vi "State XMove.vi"(6 "n":i32, 8 "error in (no error)":errorcluster, 10 "Lua to in":refnum<class "Lua.lvclass">, 11 "Lua from in":refnum<class "Lua.lvclass">) -> (0 "error out":errorcluster, 2 "Lua to out":refnum<class "Lua.lvclass">, 3 "Lua from out":refnum<class "Lua.lvclass">)   [LabVIEW 2020, in "Lua for LabVIEW.lvlib" / "Lua.lvclass"]
doc: "Starts and resumes a coroutine in the given thread L.\n\nTo start a coroutine, you push onto the thread stack the main function plus any arguments; then you call lua_resume, with nargs being the number of arguments. This call returns when the coroutine suspends or finishes its execution. When it returns, the stack contains all values passed to lua_yield, or all values returned by the body function. lua_resume returns LUA_YIELD if the coroutine yields, LUA_OK if the coroutine finishes its execution without errors, or an error code in case of errors (see lua_pcall).\n\nIn case of errors, the stack is not unwound, so you can use the debug API over it. The error object is on the top of the stack.\n\nTo resume a coroutine, you remove any results from the last lua_yield, put on its stack only the values to be passed as results from yield, and then call lua_resume.\n\nThe parameter from represents the coroutine that is resuming L. If there is no such coroutine, this parameter can be NULL."
uses:
  Lua.lvclass
  Lua.lvclass/Lua.ctl
  lib/lua.dll/lua.dll.lvlib
  lib/lua.dll/lua_thread_status.ctl
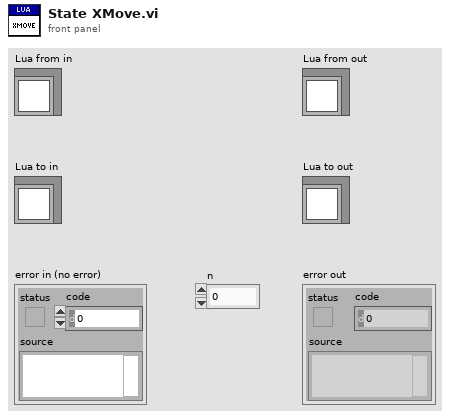
[diagram p1: front panel]
types:
  T1 = typedef "lua.dll.lvlib/lua_thread_status.ctl" = enum8{"LUA_OK", "LUA_YIELD", "LUA_ERRRUN", "LUA_ERRSYNTAX", "LUA_ERRMEM", "LUA_ERRERR"}
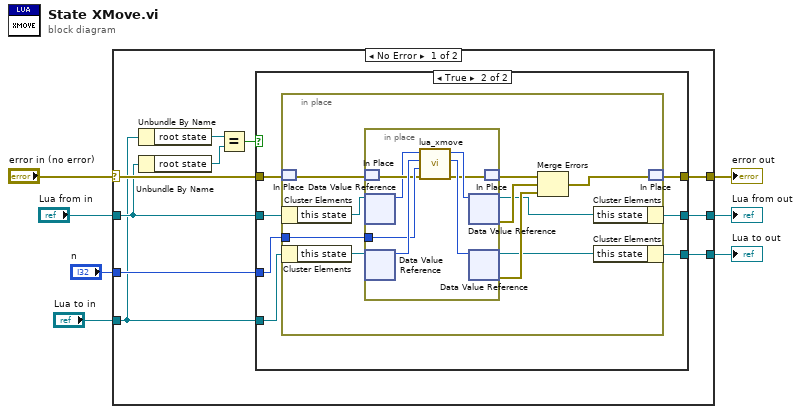
[diagram p0: block diagram]
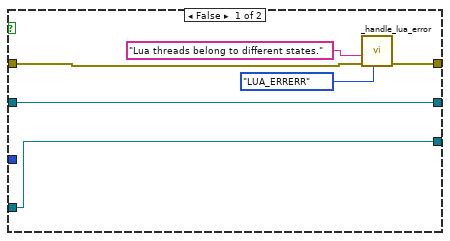
[diagram p2: hidden frame]
diagram:
  n1 = case shown="No Error" "error in (no error)" {
    selector: "error in (no error)" -> [w15 w50]
    tunnel: [w16 w50] -> w4
    tunnel: [w17 w49] -> w7
    tunnel: "Lua from in" -> [w13 w49]
    tunnel: "n" -> [w14 _]
    tunnel: "Lua to in" -> [w8 w48]
    tunnel: [w9 w48] -> w1
    frame No Error {
      n2 = Unbundle By Name(w8) -> ("root state"=w12:refnum<data-value>)
      n3 = Unbundle By Name(w13) -> ("root state"=w11:refnum<data-value>)
      n4 = Equal?(x=w12, y=w11) -> (x = y?=w10:bool)
      n5 = case shown="True" w10 {
        tunnel: [w21 w30] -> w17
        tunnel: [w22 w29] -> w16
        tunnel: w15 -> [w18 w28]
        tunnel: w14 -> [_ w27]
        tunnel: w13 -> [w21 w26]
        tunnel: [w20 w24] -> w9
        tunnel: w8 -> [w20 w25]
        frame False {
          n6 = call "_handle_lua_error.vi"("lua status"=lua_thread_status."LUA_ERRERR", "error in (no error)"=w18, "error string"="Lua threads belong to different states.") -> ("error out"=w22:errorcluster)  [unwired: 8 in]
        }
        frame True {
          n7 = in-place {
            in-place-border: w27 -> [w38]
            n8 = in-place-match #1(w28) -> (w37:errorcluster)
            n9 = in-place-cluster #2(w26) -> ("this state"=w40:refnum<data-value>)
            n10 = in-place-cluster #3(w25) -> ("this state"=w39:refnum<data-value>)
            n11 = in-place {
              in-place-border: w38 -> [w44]
              n12 = in-place-match #4(w37) -> (w43:errorcluster)
              n13 = in-place-dvr #5(w40) -> (w41:u64)  [unwired: 1 out]
              n14 = in-place-dvr #6(w39) -> (w46:u64)  [unwired: 1 out]
              n15 = call "lua_xmove.vi"("error in (no error)"=w43, "n"=w44, "to lua_state_p"=w46, "from lua_state_p"=w41) -> ("error out"=w42:errorcluster, "to lua_state_p out"=w45:u64, "from lua_state_p out"=w47:u64)  [unwired: 5 in]
              n16 = in-place-dvr #5(w47) -> (w31:refnum<data-value>, w35:errorcluster)
              n17 = in-place-dvr #6(w45) -> (w32:refnum<data-value>, w34:errorcluster)
              n18 = in-place-match #4(w42) -> (w36:errorcluster)
            }
            n19 = Merge Errors(w36, w35, w34) -> (w33:errorcluster)
            n20 = in-place-cluster #2("this state"=w31) -> (w30:refnum<class "Lua.lvclass">)
            n21 = in-place-cluster #3("this state"=w32) -> (w24:refnum<class "Lua.lvclass">)
            n22 = in-place-match #1(w33) -> (w29:errorcluster)
          }
        }
      }
    }
    frame Error {
    }
  }
  "error out" <- w4
  "Lua from out" <- w7
  "Lua to out" <- w1
